vi "File Permission Test.vi"   [LabVIEW 2017]
types:
  T1 = enum16{"open", "replace", "create", "open or create", "replace or create", "replace or create with confirmation"}
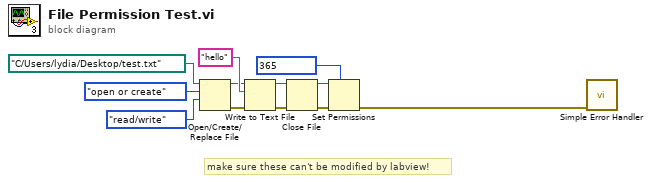
[diagram p0: block diagram]
diagram:
  # "make sure these can't be modified by labview!"
  n1 = Open/Create/Replace File(file path (use dialog)=path "C:/Users/lydia/Desktop/test.txt", operation (0:open)=T1."open or create", access (0:read/write)=enum16{"read/write", "read-only", "write-only"}."read/write") -> (refnum out=w3:refnum<file>, error out=w6:errorcluster)  [unwired: 3 in, 1 out]
  n2 = Write to Text File(file (use dialog)=w3, text="hello", error in=w6) -> (refnum out=w2:refnum<file>, error out=w5:errorcluster)  [unwired: 1 in, 1 out]
  n3 = Close File(refnum=w2, error in=w5) -> (path=w1:path, error out=w8:errorcluster)
  n4 = Set Permissions(7:i16 365 ("permissions"), 8:w8, 11:w1) -> (0:w7:errorcluster)  [unwired: 2 in, 1 out]
  n5 = call <vilib>:"Simple Error Handler.vi"("error in (no error)"=w7) -> ()  [unwired: 4 in, 5 out]
